vi "Handling DI param.vi"(5 "initialise":bool, 6 "DP":bool[](array[boolean]), 7 "connect":bool[](array[boolean]), 8 "error in (no error)":errorcluster, 9 "DI":bool[][](array[boolean]), 10 "DIP":dbl[][](array[numeric]), 11 "DI short":T1) -> (0 "error out":errorcluster, 3 "DI out":T1)   [LabVIEW 2019, in "Inputs.lvlib"]
uses:
  Inputs.lvlib
  Ctl/DI short.ctl
  Ctl/Parameter State.ctl
  DI limits calc.vi
  Logik/fronts_ext.vi
  Trigers/RS32_ext.vi
  Timer Delay/DelayR_ext.vi
  Trigers/RS_ext.vi
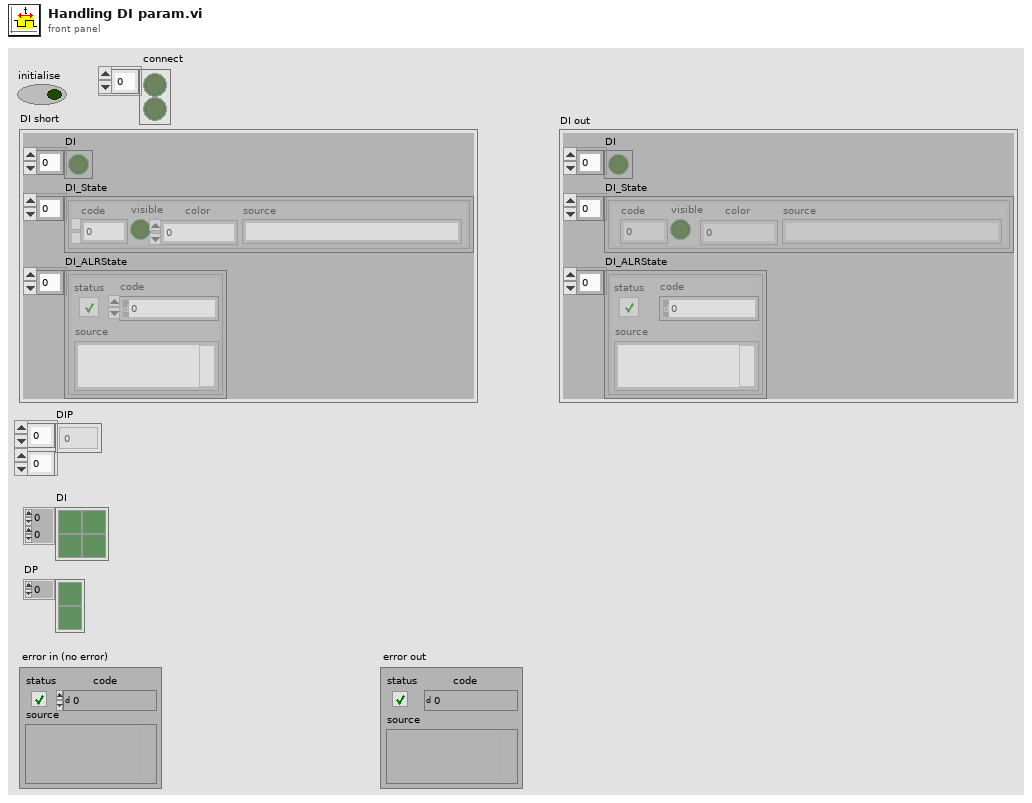
[diagram p1: front panel]
types:
  T1 = typedef "Inputs.lvlib/DI short.ctl" = cluster{"DI":bool[], "DI_State":T2[], "DI_ALRState":errorcluster[]}
  T2 = typedef "Inputs.lvlib/Parameter State.ctl" = cluster{"code":i32, "visible":bool, "color":u32, "source":string}
  T3 = cluster{"fronts not in":bool, "DelayR reg":cluster{"not in":bool, "T old":u32, "out":bool, "Q":bool}, "RS32 Q":u32}[]
  T4 = cluster{"fronts not in":bool, "DelayR reg":cluster{"not in":bool, "T old":u32, "out":bool, "Q":bool}, "RS32 Q":u32}
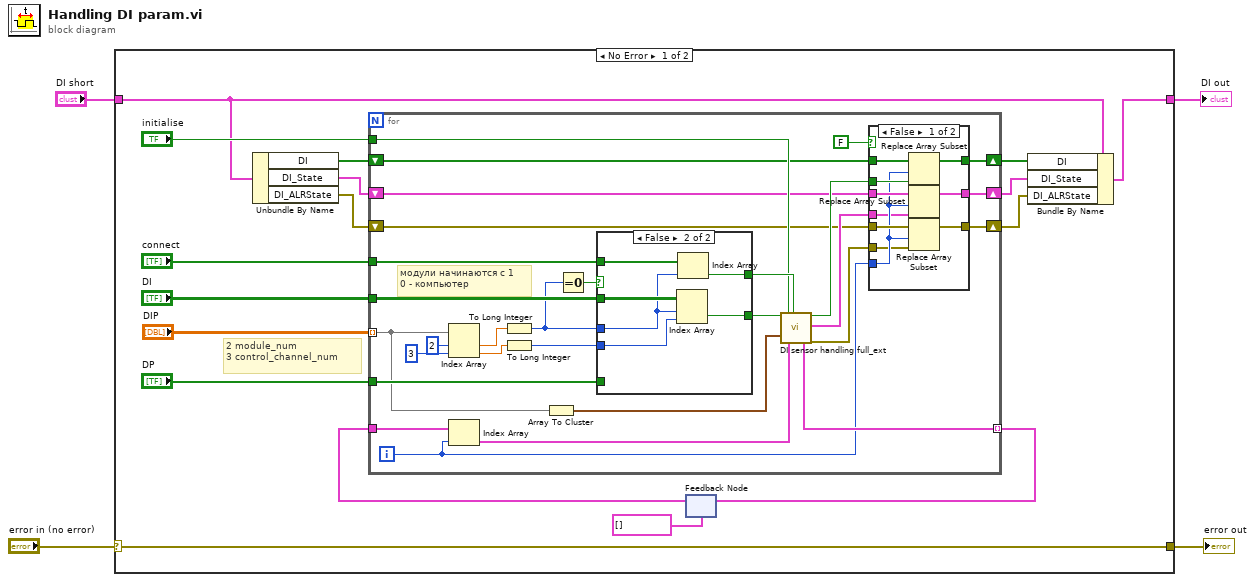
[diagram p0: block diagram]
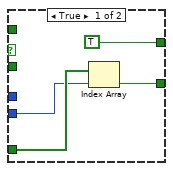
[diagram p2: hidden frame]
diagram:
  n1 = case shown="No Error" "error in (no error)" {
    selector: "error in (no error)" -> [w13 w75]
    tunnel: [w13 w75] -> w3
    tunnel: [w12 w74] -> w2
    tunnel: "DI short" -> [w5 w74]
    frame No Error {
      # "2 module_num\n3 control_channel_num"
      n2 = Unbundle By Name(w5) -> ("DI"=w11:bool[], "DI_State"=w10:T2[], "DI_ALRState"=w9:errorcluster[])
      n3 = feedback #1(T3 []) -> (w16:T3)
      n4 = for {
        tunnel: "DIP" -> [w35] mode=indexing
        tunnel: "DI" -> [w43]
        tunnel: "connect" -> [w45]
        tunnel: "initialise" -> [w32]
        tunnel: "DP" -> [w40]
        tunnel: [w31] -> w17 mode=indexing
        tunnel: w16 -> [w29]
        shift-right: [w26] -> w8
        shift-left: w11 -> [w30]
        shift-right: [w25] -> w7
        shift-left: w10 -> [w24]
        shift-right: [w22] -> w6
        shift-left: w9 -> [w23]
        i -> [w28]
        # "модули начинаются с 1\n0 - компьютер"
        n5 = Index Array(array=w35, index #1=2 ("index (col)"), index #2=3 ("index (col)")) -> (element #1=w47:dbl, element #2=w46:dbl)
        n6 = Index Array(array=w29, index=w28) -> (element=w27:T4)
        n7 = To Long Integer(number=w47) -> (32bit integer=w42:i32)
        n8 = To Long Integer(number=w46) -> (32bit integer=w41:i32)
        n9 = Array To Cluster(array=w35) -> (cluster=w34:cluster{"DIP[0]":dbl, "DIP[1]":dbl})
        n10 = Equal To 0?(x=w42) -> (x = 0?=w44:bool)
        n11 = case shown="False" w44 {
          tunnel: w43 -> [_ w60]
          tunnel: w45 -> [_ w59]
          tunnel: w42 -> [_ w57]
          tunnel: w41 -> [w53 w58]
          tunnel: w40 -> [w54 _]
          tunnel: [TRUE ("Boolean") w56] -> w39
          tunnel: [w51 w55] -> w33
          frame True {
            n12 = Index Array(array=w54, index=w53) -> (element=w51:bool)
          }
          frame False {
            n13 = Index Array(array=w60, index (row)=w57, index (col)=w58) -> (element=w55:bool)
            n14 = Index Array(array=w59, index=w57) -> (element=w56:bool)
          }
        }
        n15 = call "DI sensor handling full_ext.vi"("DI"=w33, "control"=w34, "initialise"=w32, "DI sensor handling full reg old"=w27, "connect"=w39) -> ("DI sensor handling full reg"=w31:T4, "DIOUT"=w38:bool, "STATE"=w37:T2, "ALRSTATE"=w36:errorcluster)  [unwired: 9 in, 2 out]
        n16 = case shown="False" FALSE {
          tunnel: w37 -> [w62 _]
          tunnel: w38 -> [w70 _]
          tunnel: w28 -> [w63 _]
          tunnel: w36 -> [w61 _]
          tunnel: w30 -> [w69 w73]
          tunnel: [w68 w73] -> w26
          tunnel: [w67 w71] -> w25
          tunnel: w24 -> [w66 w71]
          tunnel: w23 -> [w65 w72]
          tunnel: [w64 w72] -> w22
          frame False {
            n17 = Replace Array Subset(array=w69, new element=w70, index=w63) -> (w68:bool[])
            n18 = Replace Array Subset(array=w66, new element=w62, index=w63) -> (w67:T2[])
            n19 = Replace Array Subset(array=w65, new element=w61, index=w63) -> (w64:errorcluster[])
          }
          frame True {
          }
        }
      }
      n20 = feedback-in #1(w17) -> ()
      n21 = Bundle By Name(cluster=w5, "DI"=w8, "DI_State"=w7, "DI_ALRState"=w6) -> (w12:T1)
    }
    frame Error {
    }
  }
  "error out" <- w3
  "DI out" <- w2
